vi "BuscarPocEventoFechasNormal (SubVI).vi"(6 "Lon":string, 7 "Fecha Evento":timestamp format="%<%X\n%x>T", 8 "Lat":string, 9 "Evento":string, 10 "Imei":string, 11 "Fecha Record":timestamp format="%<%X\n%x>T") -> (1 "Query":string)   [LabVIEW 2012]
panel:
  in  "Tabla":string="Tabla1"
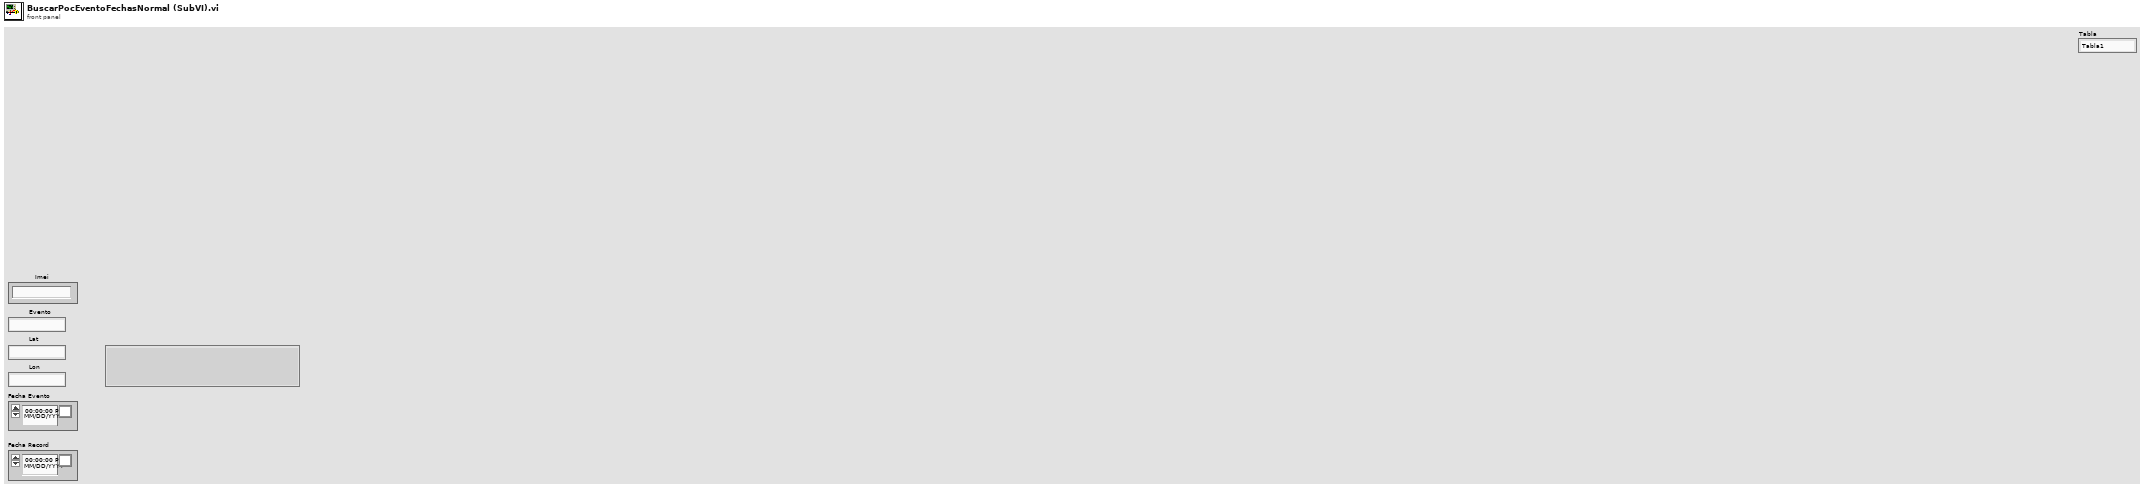
[diagram p1: front panel]
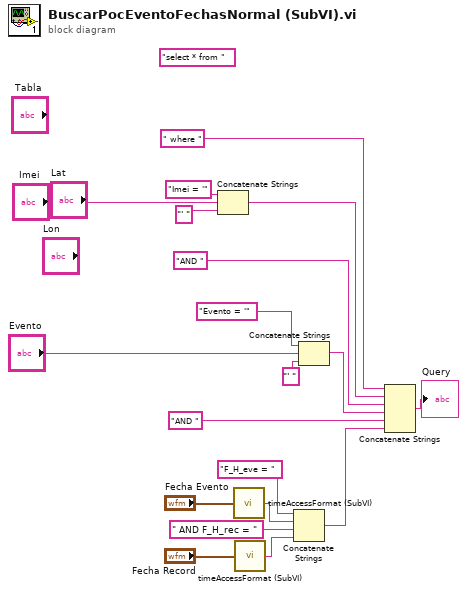
[diagram p0: block diagram]
diagram:
  (unwired) "select * from " ("SQL query")
  n1 = Concatenate Strings("Imei = '" ("Substring"), "Imei", "' " ("Substring")) -> (w13:string)
  n2 = call "timeAccessFormat (SubVI).vi"("First Date"="Fecha Evento") -> ("result string"=w5:string)
  n3 = call "timeAccessFormat (SubVI).vi"("First Date"="Fecha Record") -> ("result string"=w4:string)
  n4 = Concatenate Strings("F_H_eve = " ("string"), w5, " AND F_H_rec = " ("string"), w4) -> (w17:string)
  n5 = Concatenate Strings("Evento = '" ("string"), "Evento", "' " ("string")) -> (w18:string)
  n6 = Concatenate Strings(" where " ("Substring"), w13, "AND " ("Substring"), w18, "AND " ("Substring"), w17) -> (→"Query":string)
